vi "connect.vi"(8 "error in":errorcluster, 9 "timeout ms (5000)":i32=5000, 11 "websocket client in":refnum<class "websocket client.lvclass">) -> (0 "error out":errorcluster, 3 "websocket client out":refnum<class "websocket client.lvclass">)   [LabVIEW 2016, in "websocket client.lvclass"]
uses:
  websocket client.lvclass
  HTTP headers/http header data.ctl
  websocket client.lvclass/websocket client.ctl
  HTTP headers/http headers.lvlib
panel:
  out "headers":T1
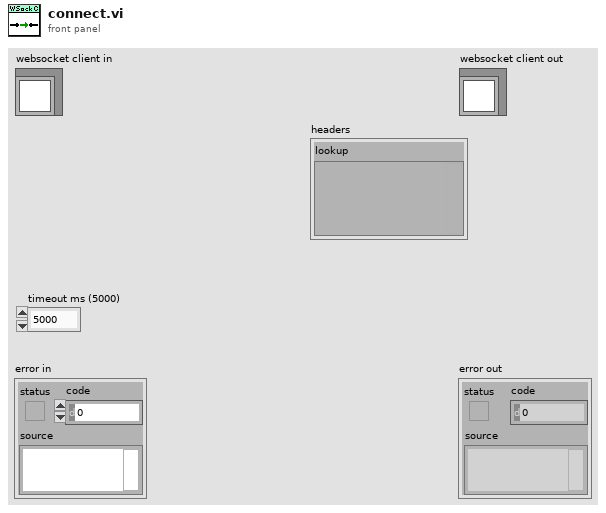
[diagram p1: front panel]
types:
  T1 = typedef "http headers.lvlib/http header data.ctl" = cluster{"lookup":variant}
  T2 = enum16{"Standard", "Buffered", "CRLF", "Immediate"}
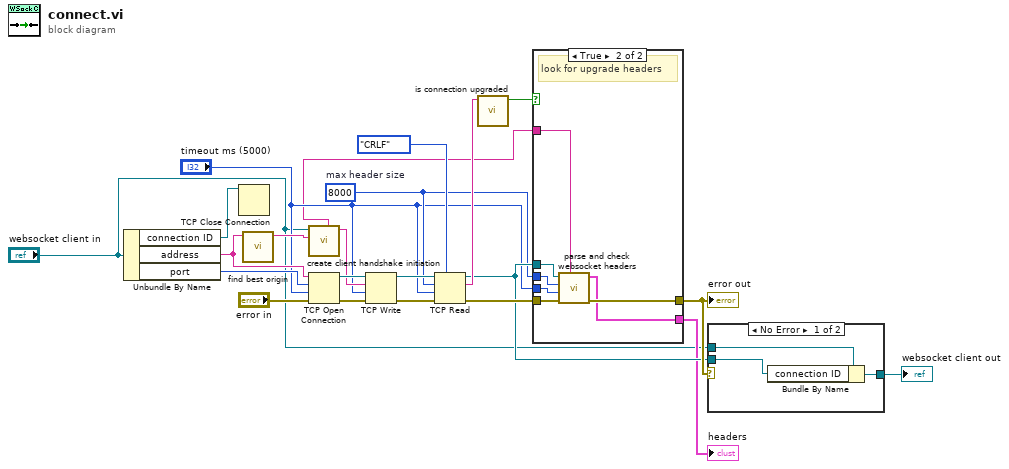
[diagram p0: block diagram]
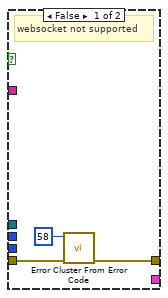
[diagram p2: hidden frame]
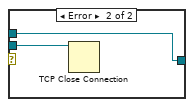
[diagram p3: hidden frame]
diagram:
  w5 = 8000  # max header size
  n1 = Unbundle By Name("websocket client in") -> ("connection ID"=w10:refnum<k5>, "address"=w9:string, "port"=w8:u16)
  n2 = TCP Close Connection(connection ID=w10) -> ()  [unwired: 2 in, 2 out]
  n3 = call "find best origin.vi"("address"=w9) -> ("origin"=w17:string)  [unwired: 10 in]
  n4 = call "create client handshake initiation.vi"("origin"=w17, "websocket client in"="websocket client in") -> ("client handshake"=w18:string, "accept key expected"=w1:string)  [unwired: 8 in]
  n5 = TCP Open Connection(address=w9, remote port or service name=w8, timeout ms (60000)="timeout ms (5000)", error in (no error)="error in") -> (connection ID=w19:refnum<k5>, error out=w7:errorcluster)  [unwired: 1 in]
  n6 = TCP Write(connection ID=w19, data in=w18, error in (no error)=w7, 9:"timeout ms (5000)") -> (connection ID out=w16:refnum<k5>, error out=w20:errorcluster)  [unwired: 1 out]
  n7 = TCP Read(connection ID=w16, bytes to read=w5, error in (no error)=w20, 7:T2."CRLF" ("mode (standard)"), 9:"timeout ms (5000)") -> (connection ID out=w6:refnum<k5>, data out=w14:string, error out=w13:errorcluster)
  n8 = call "is connection upgraded.vi"("data in"=w14) -> ("upgrade response"=w11:bool)  [unwired: 10 in]
  n9 = case shown="True" w11 {
    tunnel: w13 -> [w25 w29]
    tunnel: [w24 w28] -> w12
    tunnel: w6 -> [_ w32]
    tunnel: w5 -> [_ w31]
    tunnel: "timeout ms (5000)" -> [_ w30]
    tunnel: [_ w27] -> w3
    tunnel: w1 -> [_ w26]
    frame False {
      # "websocket not supported"
      n10 = call <vilib>:"Error Cluster From Error Code.vi"("error in (no error)"=w25, "error code (0)"=58) -> ("error out"=w24:errorcluster)  [unwired: 7 in]
    }
    frame True {
      # "look for upgrade headers"
      n11 = call "parse and check websocket headers.vi"("accept key"=w26, "error in"=w29, "timeout ms"=w30, "max header size"=w31, "TCP Network Connection in"=w32) -> ("error out"=w28:errorcluster, "headers"=w27:T1)  [unwired: 5 in]
    }
  }
  "error out" <- w12
  "headers" <- w3
  n12 = case shown="No Error" w12 {
    tunnel: [w35 w37] -> w21
    tunnel: "websocket client in" -> [w34 w37]
    tunnel: w6 -> [w33 w36]
    frame No Error {
      n13 = Bundle By Name(cluster=w34, "connection ID"=w33) -> (w35:refnum<class "websocket client.lvclass">)
    }
    frame Error {
      n14 = TCP Close Connection(connection ID=w36) -> ()  [unwired: 2 in, 2 out]
    }
  }
  "websocket client out" <- w21
